vi "read allowed execution modes.vi"(8 "error in":errorcluster, 11 "Scan Engine editor node in":refnum<class "Scan Engine editor node.lvclass">) -> (0 "error out":errorcluster, 2 "allowed execution modes":T1[](array[typedef]), 3 "Scan Engine editor node out":refnum<class "Scan Engine editor node.lvclass">)   [LabVIEW 2013, in "Scan Engine editor node.lvclass"]
uses:
  Scan Engine editor node.lvclass
  <vilib>/NI/Tag Bus Data Framework/Configuration Editor/Classes/Module editor node/Allowed Execution Modes.ctl
  <vilib>/NI/Tag Bus Data Framework/Configuration Editor/Classes/Module editor node/module editor node.lvclass
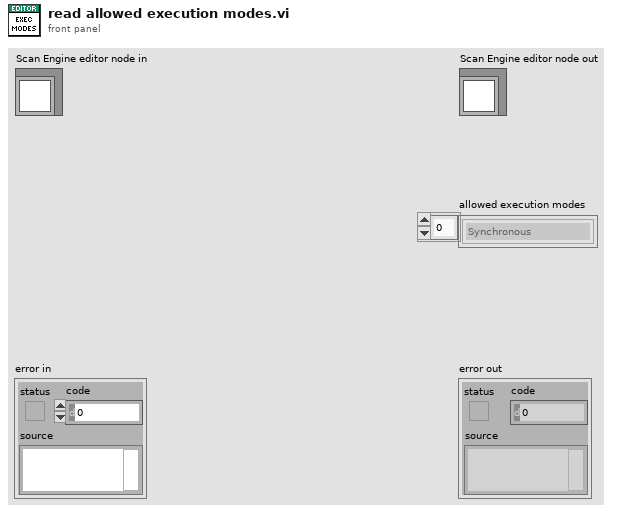
[diagram p1: front panel]
types:
  T1 = typedef "PL Framework Configuration Tool.lvlib/module editor node.lvclass/Allowed Execution Modes.ctl" = enum16{"Synchronous", "Asynchronous"}
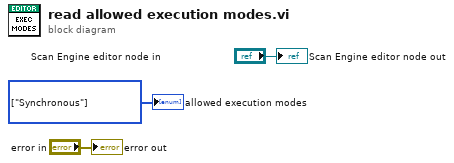
[diagram p0: block diagram]
diagram:
  w1 = T1[] [enum."Synchronous"] items=["Synchronous", "Asynchronous"] ("allowed execution modes")
  "error out" <- "error in"
  "Scan Engine editor node out" <- "Scan Engine editor node in"
  "allowed execution modes" <- w1
